vi "Mosquitto Subscriber Test.vi"() -> ()   [LabVIEW 2018]
uses:
  <vilib>/LabVIEW Open Source Project/MQTT Client/Client class/Client.lvclass/Client.ctl
  <vilib>/LabVIEW Open Source Project/MQTT Connection/MQTT_Base/Base Class/MQTT_Base.lvclass/MQTT_Base.ctl
  <vilib>/LabVIEW Open Source Project/Connection/Connection.TCP/Connection.TCP.lvclass
  C:/Program Files (x86)/National Instruments/LabVIEW 2018/vi.lib/LabVIEW Open Source Project/Connection/Connection/Connection.lvclass
  <vilib>/LabVIEW Open Source Project/MQTT Client/Client class/Client.lvclass
  C:/Program Files (x86)/National Instruments/LabVIEW 2018/vi.lib/LabVIEW Open Source Project/MQTT Connection/MQTT_Base/Base Class/MQTT_Base.lvclass
  <vilib>/LabVIEW Open Source Project/MQTT Control Packets/Control Packets/PUBLISH/PUBLISH.lvclass
  <vilib>/LabVIEW Open Source Project/MQTT Connection/MQTT_Base/Base Class/MQTT_Base.lvclass
  <vilib>/LabVIEW Open Source Project/Connection/Connection.LocalQueue/Connection.LocalQueue.lvclass
  <vilib>/LabVIEW Open Source Project/Connection/Connection/Connection.lvclass
panel:
  out "Suback 2":bool
  out "Unsuback 2":bool
  in  "text Subscribe":bool
  in  "Topic Name":string="$SYS/#"
  in  "broker address":string(combo)="test.mosquitto.org"
  out "string":string
  out "Payload":u8[](array[numeric]) format="%08b"
  out "Topic":string
  out "Unsuback":bool
  out "Suback":bool
  in  "Subscribe":bool
  in  "Connection":bool
  in  "Stop Client":bool
  out "Waveform Chart":dbl(graph)
  out "last error":errorcluster
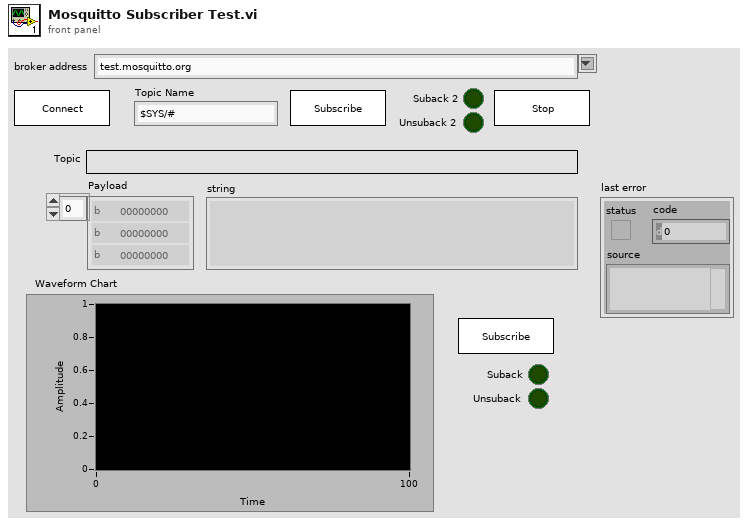
[diagram p1: front panel]
types:
  T1 = typedef "MQTT Client.lvlib/Client.lvclass/Public Events -- cluster.ctl" = cluster{"Connection Status":refnum<user-event>, "Connected":refnum<user-event>, "Application Message":refnum<user-event>}
  T2 = typedef "MQTT Base.lvlib/MQTT_Base.lvclass/Public Events -- cluster.ctl" = cluster{"Stop Event":refnum<user-event>, "Error Event":refnum<user-event>, "Inbound Message":refnum<user-event>}
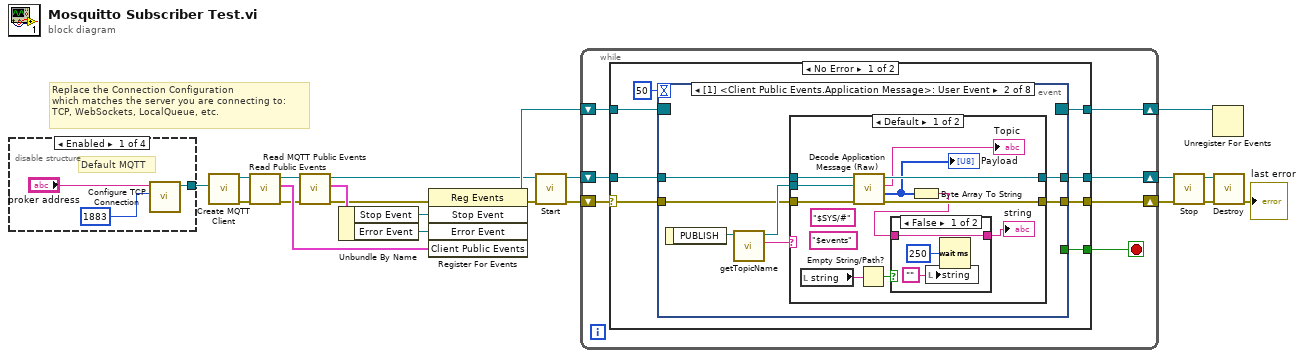
[diagram p0: block diagram]
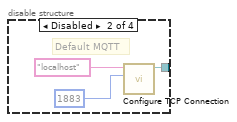
[diagram p2: hidden frame]
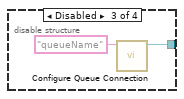
[diagram p3: hidden frame]
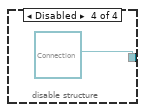
[diagram p4: hidden frame]
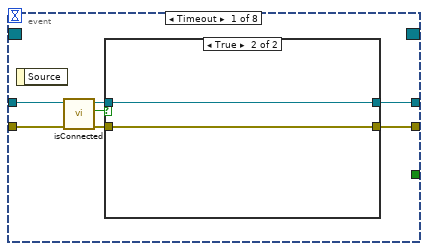
[diagram p5: hidden frame]
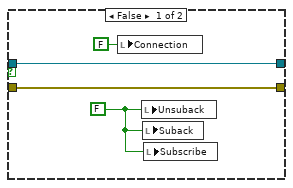
[diagram p6: hidden frame]
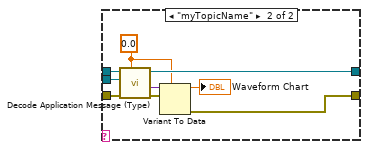
[diagram p8: hidden frame]
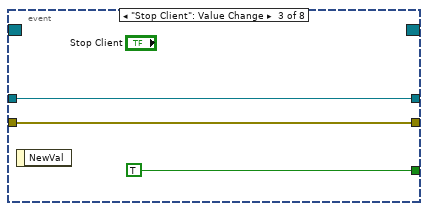
[diagram p9: hidden frame]
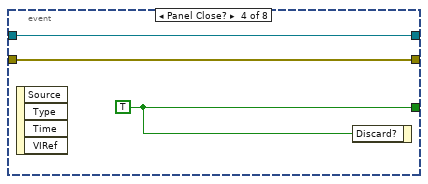
[diagram p10: hidden frame]
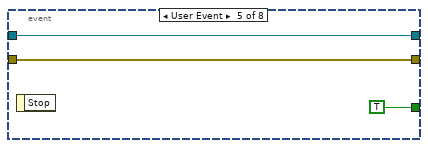
[diagram p11: hidden frame]
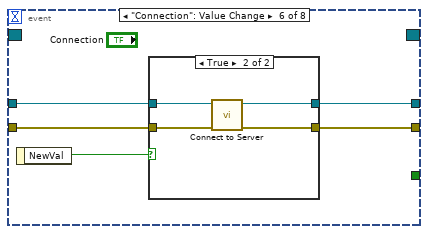
[diagram p12: hidden frame]
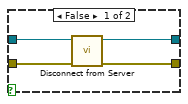
[diagram p13: hidden frame]
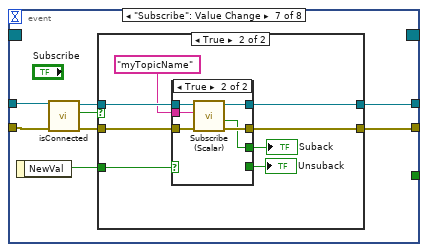
[diagram p14: hidden frame]
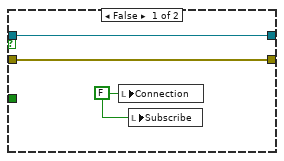
[diagram p15: hidden frame]
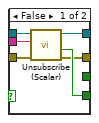
[diagram p16: hidden frame]
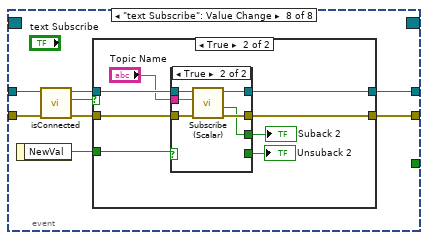
[diagram p17: hidden frame]
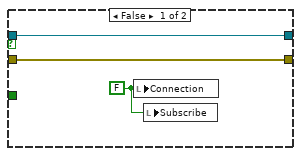
[diagram p18: hidden frame]
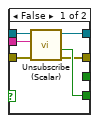
[diagram p19: hidden frame]
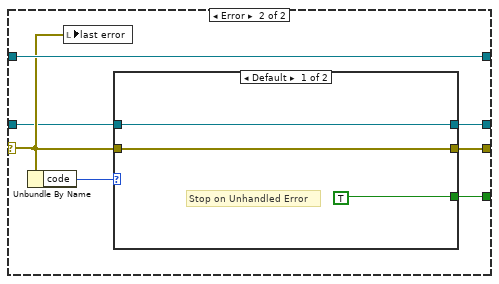
[diagram p20: hidden frame]
diagram:
  # "Replace the Connection Configuration\nwhich matches the server you are connecting to:\nTCP, WebSockets, LocalQueue, etc."
  n1 = disable-structure shown="Enabled" {
    disable-tunnel: [w23 w26 w29 refnum<class "Connection.lvclass"> refnum ("Connection Configuration")] -> w21
    frame Enabled {
      # "Default MQTT"
      n2 = call <vilib>:"Configure TCP Connection.vi"("remote port (80)"=u16 1883, "address (localhost)"="broker address") -> ("Connection.TCP"=w23:refnum<class "Connection.TCP.lvclass">)  [unwired: 8 in, 1 out]
    }
    frame Disabled {
      # "Default MQTT"
      n3 = call <vilib>:"Configure TCP Connection.vi"("remote port (80)"=u16 1883, "address (localhost)"="localhost") -> ("Connection.TCP"=w26:refnum<class "Connection.TCP.lvclass">)  [unwired: 8 in, 1 out]
    }
    frame Disabled {
      n4 = call <vilib>:"Configure Queue Connection.vi"("Queue Name"="queueName") -> ("Connection.LocalQueue"=w29:refnum<class "Connection.LocalQueue.lvclass">)  [unwired: 9 in, 1 out]
    }
    frame Disabled {
    }
  }
  n5 = call <vilib>:"Create MQTT Client.vi"("Connection Configuration"=w21) -> ("error out"=w3:errorcluster, "Client out"=w1:refnum<class "Client.lvclass">)  [unwired: 9 in]
  n6 = call <vilib>:"Read Public Events.vi"("error in (no error)"=w3, "Client in"=w1) -> ("error out"=w4:errorcluster, "Client Public Events"=w6:T1, "Client out"=w2:refnum<class "Client.lvclass">)  [unwired: 7 in]
  n7 = call <vilib>:"Read MQTT Public Events.vi"("error in (no error)"=w4, "MQTT_Base in"=w2) -> ("error out"=w5:errorcluster, "MQTT Public Events"=w13:T2, "MQTT_Base out"=w8:refnum<class "Client.lvclass">)  [unwired: 7 in]
  n8 = Unbundle By Name(w13) -> ("Stop Event"=w11:refnum<user-event>, "Error Event"=w12:refnum<user-event>)
  n9 = register-events(error in=w5, w11, w12, w6) -> (reference out=w9:refnum<event-registration>, error out=w7:errorcluster)  [unwired: 1 in]
  n10 = call <vilib>:"Start.vi"("error in (no error)"=w7, "MQTT_Base in"=w8) -> ("error out"=w19:errorcluster, "MQTT_Base out"=w18:refnum<class "Client.lvclass">)  [unwired: 7 in, 1 out]
  n11 = while {
    shift-right: [w36] -> w10
    shift-left: w9 -> [w37]
    shift-right: [w33] -> w15
    shift-left: w18 -> [w34]
    shift-right: [w35] -> w17
    shift-left: w19 -> [w31]
    stop <- w32 stop-if-true
    n12 = case shown="No Error" w31 {
      selector: w31 -> [w38 w177]
      tunnel: w37 -> [w45 w180]
      tunnel: [w44 w180] -> w36
      tunnel: [w43 w175] -> w35
      tunnel: w34 -> [w41 w176]
      tunnel: [w40 w179] -> w33
      tunnel: [w39 w174] -> w32
      frame No Error {
        n13 = event shown="[1] <Client Public Events.Application Message>: User Event" {
          selector: w45 -> [_ _ _ _ _ _ _ _]
          dyn-events: [_ _ _ _ _ _ _ _] -> w44
          timeout: 50 -> [_ _ _ _ _ _ _ _]
          tunnel: w38 -> [w48 w62 w91 w93 w98 w99 w117 w149]
          tunnel: [w51 w59 w91 w93 w98 w100 w118 w145] -> w43
          tunnel: [_ _ TRUE w95 TRUE _ _ _] -> w39
          tunnel: w41 -> [w50 w63 w92 w94 w96 w103 w116 w150]
          tunnel: [w52 w61 w92 w94 w96 w101 w119 w144] -> w40
          event Timeout {
            n14 = event-data() -> ()  [unwired: 1 in, 1 out]
            n15 = call <vilib>:"isConnected.vi"("error in (no error)"=w48, "Client in"=w50) -> ("error out"=w47:errorcluster, "connected"=w46:bool, "Client out"=w49:refnum<class "Client.lvclass">)  [unwired: 7 in]
            n16 = case shown="True" w46 {
              tunnel: [w56 w58] -> w52
              tunnel: [w55 w57] -> w51
              tunnel: w49 -> [w56 w58]
              tunnel: w47 -> [w55 w57]
              frame False {
                w54 = FALSE
                n17 = local write "Connection"(FALSE ("Connection")) -> ()
                n18 = local write "Unsuback"(w54) -> ()
                n19 = local write "Suback"(w54) -> ()
                n20 = local write "Subscribe"(w54) -> ()
              }
              frame True {
              }
            }
          }
          event User Event {
            n21 = event-data() -> ("PUBLISH"=w65:refnum<class "PUBLISH.lvclass">)  [unwired: 1 in]
            n22 = call <vilib>:"getTopicName.vi"("PUBLISH in"=w65) -> ("Topic"=w60:string, "PUBLISH out"=w64:refnum<class "PUBLISH.lvclass">)  [unwired: 8 in, 1 out]
            n23 = case shown="Default" w60 {
              tunnel: w64 -> [w70 w81]
              tunnel: w63 -> [w76 w87]
              tunnel: w62 -> [w75 w85]
              tunnel: [w73 w86] -> w61
              tunnel: [w74 w89] -> w59
              frame Default {
                (unwired) "$events"
                (unwired) "$SYS/#" ("Topic Name")
                n24 = local read "string"() -> (w69:string)
                n25 = call <vilib>:"Decode Application Message (Raw).vi"("error in (no error)"=w75, "PUBLISH"=w70, "Client in"=w76) -> ("error out"=w74:errorcluster, "Payload"=w71:u8[], "Topic"=→"Topic":string, "Client out"=w73:refnum<class "Client.lvclass">)  [unwired: 5 in]
                "Payload" <- w71
                n26 = Empty String/Path?(string/path=w69) -> (empty?=w68:bool)
                n27 = Byte Array To String(unsigned byte array=w71) -> (string=w67:string)
                n28 = case shown="False" w68 {
                  tunnel: w67 -> [w78 w80]
                  tunnel: [w78 w80] -> w66
                  frame False {
                    n29 = local write "string"("") -> ()
                    n30 = Wait (ms)(milliseconds to wait=u32 250) -> ()  [unwired: 1 out]
                  }
                  frame True {
                  }
                }
                "string" <- w66
              }
              frame "myTopicName" {
                w83 = 0.0
                n31 = call <vilib>:"Decode Application Message (Type).vi"("Type"=w83, "error in (no error)"=w85, "PUBLISH"=w81, "Client in"=w87) -> ("error out"=w84:errorcluster, "Payload"=w82:variant, "Client out"=w86:refnum<class "Client.lvclass">)  [unwired: 4 in, 1 out]
                n32 = Variant To Data(error in=w84, type=w83, Variant=w82) -> (data=→"Waveform Chart":dbl, error out=w89:errorcluster)
              }
            }
          }
          event "Stop Client": Value Change {
            n33 = event-data() -> ()  [unwired: 1 in, 1 out]
          }
          event Panel Close? {
            w95 = TRUE
            n34 = event-data() -> ()  [unwired: 1 in, 4 out]
            n35 = event-data("Discard?"=w95) -> ()  [unwired: 1 in, 1 out]
          }
          event User Event {
            n36 = event-data() -> ()  [unwired: 1 in, 1 out]
          }
          event "Connection": Value Change {
            n37 = event-data() -> ("NewVal"=w102:bool)  [unwired: 1 in]
            n38 = case shown="True" w102 {
              tunnel: w103 -> [w107 w111]
              tunnel: [w106 w108] -> w101
              tunnel: [w105 w109] -> w100
              tunnel: w99 -> [w104 w110]
              frame False {
                n39 = call <vilib>:"Disconnect from Server.vi"("error in (no error)"=w104, "Client in"=w107) -> ("error out"=w105:errorcluster, "Client out"=w106:refnum<class "Client.lvclass">)  [unwired: 7 in, 1 out]
              }
              frame True {
                n40 = call <vilib>:"Connect to Server.vi"("error in (no error)"=w110, "Client in"=w111) -> ("error out"=w109:errorcluster, "Client out"=w108:refnum<class "Client.lvclass">)  [unwired: 6 in, 2 out]
              }
            }
          }
          event "Subscribe": Value Change {
            n41 = event-data() -> ("NewVal"=w112:bool)  [unwired: 1 in]
            n42 = call <vilib>:"isConnected.vi"("error in (no error)"=w117, "Client in"=w116) -> ("error out"=w114:errorcluster, "connected"=w113:bool, "Client out"=w115:refnum<class "Client.lvclass">)  [unwired: 7 in]
            n43 = case shown="True" w113 {
              tunnel: [w122 w130] -> w119
              tunnel: [w121 w129] -> w118
              tunnel: w115 -> [w122 w128]
              tunnel: w114 -> [w121 w127]
              tunnel: w112 -> [_ w126]
              frame False {
                w120 = FALSE ("Connection")
                n44 = local write "Connection"(w120) -> ()
                n45 = local write "Subscribe"(w120) -> ()
              }
              frame True {
                n46 = case shown="True" w126 {
                  tunnel: [w131 w139] -> w130
                  tunnel: [w132 w138] -> w129
                  tunnel: w128 -> [w136 w142]
                  tunnel: w127 -> [w135 w141]
                  tunnel: "myTopicName" ("Topic Name (empty: Payload name)") -> [w134 w140]
                  tunnel: [_ w137] -> w125
                  tunnel: [w133 _] -> w124
                  frame False {
                    n47 = call <vilib>:"Unsubscribe (Scalar).vi"("error in (no error)"=w135, "Topic Filter"=w134, "Client in"=w136) -> ("error out"=w132:errorcluster, "Ack"=w133:bool, "Client out"=w131:refnum<class "Client.lvclass">)  [unwired: 6 in]
                  }
                  frame True {
                    n48 = call <vilib>:"Subscribe (Scalar).vi"("error in (no error)"=w141, "Topic Filter"=w140, "Client in"=w142) -> ("error out"=w138:errorcluster, "Ack"=w137:bool, "Client out"=w139:refnum<class "Client.lvclass">)  [unwired: 6 in]
                  }
                }
                "Unsuback" <- w124
                "Suback" <- w125
              }
            }
          }
          event "text Subscribe": Value Change {
            n49 = event-data() -> ("NewVal"=w143:bool)  [unwired: 1 in]
            n50 = call <vilib>:"isConnected.vi"("error in (no error)"=w149, "Client in"=w150) -> ("error out"=w146:errorcluster, "connected"=w148:bool, "Client out"=w147:refnum<class "Client.lvclass">)  [unwired: 7 in]
            n51 = case shown="True" w148 {
              tunnel: w147 -> [w151 w160]
              tunnel: w146 -> [w152 w161]
              tunnel: [w152 w156] -> w145
              tunnel: [w151 w155] -> w144
              tunnel: w143 -> [_ w154]
              frame False {
                w153 = FALSE ("Connection")
                n52 = local write "Connection"(w153) -> ()
                n53 = local write "Subscribe"(w153) -> ()
              }
              frame True {
                n54 = case shown="True" w154 {
                  tunnel: [w162 w170] -> w155
                  tunnel: [w163 w169] -> w156
                  tunnel: w160 -> [w167 w173]
                  tunnel: w161 -> [w166 w172]
                  tunnel: "Topic Name" -> [w165 w171]
                  tunnel: [_ w168] -> w158
                  tunnel: [w164 _] -> w157
                  frame False {
                    n55 = call <vilib>:"Unsubscribe (Scalar).vi"("error in (no error)"=w166, "Topic Filter"=w165, "Client in"=w167) -> ("error out"=w163:errorcluster, "Ack"=w164:bool, "Client out"=w162:refnum<class "Client.lvclass">)  [unwired: 6 in]
                  }
                  frame True {
                    n56 = call <vilib>:"Subscribe (Scalar).vi"("error in (no error)"=w172, "Topic Filter"=w171, "Client in"=w173) -> ("error out"=w169:errorcluster, "Ack"=w168:bool, "Client out"=w170:refnum<class "Client.lvclass">)  [unwired: 6 in]
                  }
                }
                "Unsuback 2" <- w157
                "Suback 2" <- w158
              }
            }
          }
        }
      }
      frame Error {
        n57 = Unbundle By Name(w177) -> ("code"=w178:i32)
        n58 = local write "last error"(w177) -> ()
        n59 = case shown="Default" w178 {
          tunnel: w176 -> [w183 w184]
          tunnel: [w183 w184] -> w179
          tunnel: w177 -> [w182 _]
          tunnel: [w182 _] -> w175
          tunnel: [TRUE _] -> w174
          frame Default {
            # "Stop on Unhandled Error"
          }
          frame 56, 63, 66 {
            # "Disconnected"
          }
        }
      }
    }
  }
  n60 = call <vilib>:"Stop.vi"("error in (no error)"=w17, "MQTT_Base in"=w15) -> ("error out"=w16:errorcluster, "MQTT_Base out"=w14:refnum<class "Client.lvclass">)  [unwired: 7 in, 1 out]
  n61 = Unregister For Events(event registration refnum=w10) -> ()  [unwired: 1 in, 1 out]
  n62 = call <vilib>:"Destroy.vi"("error in (no error)"=w16, "MQTT_Base in"=w14) -> ("error out"=→"last error":errorcluster)  [unwired: 8 in, 1 out]
